vi "log analysis_gps.vi"() -> ()   [LabVIEW 2019] (continued)
\tsystem status\tnormal 2 27.800000 0 0\trobot status\t31.327624\t41.295864\t9.189700\t-0.525200\t0.456230\t-124.593983\t0.494000\t-0.009000\n\t\n15:51:51.4\tlog_raw\tgps_raw\t#INSPVAXA,USB3,0,48.0,FINESTEERING,2107,283929.450,02000000,471d,15824;INS_ALIGNMENT_COMPLETE,INS_RTKFIXED,37.37050057739,126.72118712143,9.1936,22.3000,-0.3554,-0.3037,0.0227,-0.396145969,0.312216334,214.731264498,0.4324,0.3037,0.5892,0.1125,0.0933,0.0800,0.0956,0.0998,5.2109,0f000001,0*e8b24b74\n\tsystem status\tnormal 2 27.800000 0 0\trobot status\t31.181031\t41.106514\t9.193600\t-0.396146\t0.312216\t-124.731264\t0.495000\t-0.003000\n\t\n15:51:51.9\tlog_raw\tgps_raw\t#INSPVAXA,USB3,0,48.0,FINESTEERING,2107,283929.950,02000000,471d,15824;INS_ALIGNMENT_COMPLETE,INS_RTKFIXED,37.37049890881,126.72118550326,9.1969,22.3000,-0.3488,-0.2994,0.0296,-0.491904024,0.536179959,214.904903866,0.4324,0.3037,0.5892,0.1125,0.0933,0.0800,0.0956,0.0998,5.2109,0f000001,0*ad87a7a5\n\tsystem status\tnormal 2 27.800000 0 0\trobot status\t31.037696\t40.921328\t9.196900\t-0.491904\t0.536180\t-124.904904\t0.491000\t-0.006000\n\t\n15:51:52.4\tlog_raw\tgps_raw\t#INSPVAXA,USB3,0,48.5,FINESTEERING,2107,283930.450,02000000,471d,15824;INS_ALIGNMENT_COMPLETE,INS_RTKFIXED,37.37049721050,126.72118386884,9.1995,22.3000,-0.3636,-0.2994,0.0018,-0.629398853,0.403170896,215.071222614,0.4325,0.3033,0.5894,0.1129,0.0937,0.0807,0.0956,0.0998,5.2121,0f000001,0*cd026204\n\tsystem status\tnormal 2 27.800000 0 0\trobot status\t30.892922\t40.732842\t9.199500\t-0.629399\t0.403171\t-125.071223\t0.499000\t-0.003000\n\t\n15:51:52.9\tlog_raw\tgps_raw\t#INSPVAXA,USB3,0,48.5,FINESTEERING,2107,283930.950,02000000,471d,15824;INS_ALIGNMENT_COMPLETE,INS_RTKFIXED,37.37049554136,126.72118223903,9.2033,22.3000,-0.3579,-0.3114,0.0267,-0.630465931,0.456383664,215.164754622,0.4325,0.3033,0.5894,0.1129,0.0937,0.0807,0.0956,0.0998,5.2121,0f000001,0*d7b4217a\n\tsystem status\tnormal 2 27.800000 0 0\trobot status\t30.748556\t40.547594\t9.203300\t-0.630466\t0.456384\t-125.164755\t0.497000\t-0.001000\n\t\n15:51:53.4\tlog_raw\tgps_raw\t#INSPVAXA,USB3,0,51.0,FINESTEERING,2107,283931.450,02000000,471d,15824;INS_ALIGNMENT_COMPLETE,INS_RTKFIXED,37.37049384282,126.72118058399,9.2075,22.3000,-0.3544,-0.2989,0.0161,-0.740038291,0.456521512,215.355756173,0.4326,0.3033,0.5897,0.1135,0.0944,0.0819,0.0956,0.0998,5.2130,0f000001,0*1b20caf7\n\tsystem status\tnormal 2 27.800000 0 0\trobot status\t30.601955\t40.359083\t9.207500\t-0.740038\t0.456522\t-125.355756\t0.493000\t-0.002000\n\t\n15:51:53.9\tlog_raw\tgps_raw\t#INSPVAXA,USB3,0,51.0,FINESTEERING,2107,283931.950,02000000,471d,15824;INS_ALIGNMENT_COMPLETE,INS_RTKFIXED,37.37049213218,126.72117889345,9.2111,22.3000,-0.3596,-0.3121,0.0183,-0.657813953,0.413680306,215.408958644,0.4326,0.3033,0.5897,0.1135,0.0944,0.0819,0.0956,0.0998,5.2130,0f000001,0*a46484af\n\tsystem status\tnormal 2 27.800000 0 0\trobot status\t30.452210\t40.169228\t9.211100\t-0.657814\t0.413680\t-125.408959\t0.501000\t0.009000\n\t\n15:51:54.4\tlog_raw\tgps_raw\t#INSPVAXA,USB3,0,50.0,FINESTEERING,2107,283932.450,02000000,471d,15824;INS_ALIGNMENT_COMPLETE,INS_RTKFIXED,37.37049046733,126.72117722659,9.2158,22.3000,-0.3473,-0.3092,0.0349,-0.590608670,0.319388706,215.361013781,0.4329,0.3036,0.5903,0.1143,0.0953,0.0834,0.0957,0.0998,5.2135,0f000001,0*5573a11c\n\tsystem status\tnormal 2 27.800000 0 0\trobot status\t30.304562\t39.984456\t9.215800\t-0.590609\t0.319389\t-125.361014\t0.489000\t0.004000\n\t\n15:51:54.9\tlog_raw\tgps_raw\t#INSPVAXA,USB3,0,50.0,FINESTEERING,2107,283932.950,02000000,471d,15824;INS_ALIGNMENT_COMPLETE,INS_RTKFIXED,37.37048877805,126.72117553421,9.2224,22.3000,-0.3576,-0.3071,0.0334,-0.545773763,0.550162659,215.419033819,0.4329,0.3036,0.5903,0.1143,0.0953,0.0834,0.0957,0.0998,5.2135,0f000001,0*06d0156c\n\tsystem status\tnormal 2 27.800000 0 0\trobot status\t30.154654\t39.796973\t9.222400\t-0.545774\t0.550163\t-125.419034\t0.505000\t-0.004000\n\t\n15:51:55.4\tlog_raw\tgps_raw\t#INSPVAXA,USB3,0,46.5,FINESTEERING,2107,283933.450,02000000,471d,15824;INS_ALIGNMENT_COMPLETE,INS_RTKFIXED,37.37048709327,126.72117385484,9.2273,22.3000,-0.3583,-0.3032,0.0201,-0.584226709,0.709789470,215.528367136,0.4335,0.3040,0.5913,0.1137,0.0945,0.0830,0.0957,0.0998,5.2139,0f000001,0*ba7d8e29\n\tsystem status\tnormal 2 27.800000 0 0\trobot status\t30.005898\t39.609989\t9.227300\t-0.584227\t0.709789\t-125.528367\t0.492000\t-0.004000\n\t\n15:51:55.9\tlog_raw\tgps_raw\t#INSPVAXA,USB3,0,46.5,FINESTEERING,2107,283933.950,02000000,471d,15824;INS_ALIGNMENT_COMPLETE,INS_RTKFIXED,37.37048540421,126.72117215519,9.2325,22.3000,-0.3686,-0.3092,0.0093,-0.663238373,0.676190653,215.463359493,0.4335,0.3040,0.5913,0.1137,0.0945,0.0830,0.0957,0.0998,5.2139,0f000001,0*5a7d9a35\n\tsystem status\tnormal 2 27.800000 0 0\trobot status\t29.855346\t39.422530\t9.232500\t-0.663238\t0.676191\t-125.463359\t0.494000\t0.014000\n\t\n15:51:56.4\tlog_raw\tgps_raw\t#INSPVAXA,USB3,0,51.5,FINESTEERING,2107,283934.450,02000000,471d,15824;INS_ALIGNMENT_COMPLETE,INS_RTKFIXED,37.37048375352,126.72117048246,9.2375,22.3000,-0.3734,-0.3205,0.0340,-0.435969106,0.945574003,215.391049185,0.4334,0.3041,0.5920,0.1131,0.0939,0.0826,0.0958,0.0998,5.2143,0f000001,0*bcbd8a70\n\tsystem status\tnormal 2 27.700000 0 0\trobot status\t29.707178\t39.239329\t9.237500\t-0.435969\t0.945574\t-125.391049\t0.482000\t0.004000\n\t\n15:51:56.9\tlog_raw\tgps_raw\t#INSPVAXA,USB3,0,51.5,FINESTEERING,2107,283934.950,02000000,471d,15824;INS_ALIGNMENT_COMPLETE,INS_RTKFIXED,37.37048205847,126.72116880230,9.2433,22.3000,-0.3752,-0.3030,0.0191,-0.551123480,0.797684003,215.136467002,0.4334,0.3041,0.5920,0.1131,0.0939,0.0826,0.0958,0.0998,5.2143,0f000001,0*2d6be551\n\tsystem status\tnormal 2 27.700000 0 0\trobot status\t29.558352\t39.051205\t9.243300\t-0.551123\t0.797684\t-125.136467\t0.596000\t-0.155000\n\t\n15:51:57.4\tlog_raw\tgps_raw\t\tsystem status\tnormal 2 27.700000 0 0\trobot status\t29.409840\t38.862241\t9.248200\t-0.605044\t0.730671\t-124.996837\t0.601000\t-0.133000\n\t\n15:51:57.9\tlog_raw\tgps_raw\t#INSPVAXA,USB3,0,49.0,FINESTEERING,2107,283935.950,02000000,471d,15824;INS_ALIGNMENT_COMPLETE,INS_RTKFIXED,37.37047866137,126.72116545098,9.2537,22.3000,-0.3697,-0.3129,0.0257,-0.409292319,0.632531125,214.781702011,0.4334,0.3038,0.5927,0.1127,0.0935,0.0821,0.0959,0.0999,5.2145,0f000001,0*763cf472\n\tsystem status\tnormal 2 27.700000 0 0\trobot status\t29.261498\t38.674180\t9.253700\t-0.409292\t0.632531\t-124.781702\t0.607000\t-0.165000\n\t\n15:51:58.4\tlog_raw\tgps_raw\t#INSPVAXA,USB3,0,48.0,FINESTEERING,2107,283936.450,02000000,471d,15824;INS_ALIGNMENT_COMPLETE,INS_RTKFIXED,37.37047695933,126.72116379842,9.2575,22.3000,-0.3601,-0.2905,0.0223,-0.510166928,0.275357051,214.549267942,0.4332,0.3032,0.5933,0.1122,0.0932,0.0817,0.0960,0.0999,5.2143,0f000001,0*907ae007\n\tsystem status\tnormal 2 27.800000 0 0\trobot status\t29.115117\t38.485281\t9.257500\t-0.510167\t0.275357\t-124.549268\t0.469000\t0.034000\n\t\n15:51:58.9\tlog_raw\tgps_raw\t#INSPVAXA,USB3,0,48.0,FINESTEERING,2107,283936.950,02000000,471d,15824;INS_ALIGNMENT_COMPLETE,INS_RTKFIXED,37.37047527853,126.72116215716,9.2617,22.3000,-0.3613,-0.3073,0.0319,-0.493749348,0.435637715,214.244212344,0.4332,0.3032,0.5933,0.1122,0.0932,0.0817,0.0960,0.0999,5.2143,0f000001,0*77c5d1d8\n\tsystem status\tnormal 2 27.700000 0 0\trobot status\t28.969737\t38.298738\t9.261700\t-0.493749\t0.435638\t-124.244212\t0.497000\t-0.002000\n\t\n15:51:59.4\tlog_raw\tgps_raw\t\tsystem status\tnormal 2 27.700000 0 0\trobot status\t28.825588\t38.110134\t9.265500\t-0.511173\t0.534188\t-124.033120\t0.472000\t0.046000\n\t\n15:51:59.9\tlog_raw\tgps_raw\t#INSPVAXA,USB3,0,48.5,FINESTEERING,2107,283937.950,02000000,471d,15824;INS_ALIGNMENT_COMPLETE,INS_RTKFIXED,37.37047189710,126.72115890646,9.2688,22.3000,-0.3586,-0.2934,0.0244,-0.533486904,0.671561834,213.833990455,0.4328,0.3028,0.5937,0.1126,0.0939,0.0822,0.0961,0.1000,5.2146,0f000001,0*9215f66d\n\tsystem status\tnormal 2 27.700000 0 0\trobot status\t28.681795\t37.923453\t9.268800\t-0.533487\t0.671562\t-123.833990\t0.581000\t-0.140000\n\t\n15:52:00.4\tlog_raw\tgps_raw\t#INSPVAXA,USB3,0,52.0,FINESTEERING,2107,283938.450,02000000,471d,15824;INS_ALIGNMENT_COMPLETE,INS_RTKFIXED,37.37047020437,126.72115727420,9.2725,22.3000,-0.3547,-0.3143,0.0241,-0.356445317,0.659835202,213.629028548,0.4325,0.3026,0.5940,0.1125,0.0937,0.0818,0.0961,0.1000,5.2151,0f000001,0*9a205bce\n\tsystem status\tnormal 2 27.700000 0 0\trobot status\t28.537212\t37.735586\t9.272500\t-0.356445\t0.659835\t-123.629029\t0.583000\t-0.116000\n\t\n15:52:00.9\tlog_raw\tgps_raw\t#INSPVAXA,USB3,0,52.0,FINESTEERING,2107,283938.950,02000000,471d,15824;INS_ALIGNMENT_COMPLETE,INS_RTKFIXED,37.37046851551,126.72115567512,9.2776,22.3000,-0.3685,-0.3042,0.0189,-0.419579821,0.629946557,213.500724202,0.4325,0.3026,0.5940,0.1125,0.0937,0.0818,0.0961,0.1000,5.2151,0f000001,0*4752d92c\n\tsystem status\tnormal 2 27.700000 0 0\trobot status\t28.395568\t37.548149\t9.277600\t-0.419580\t0.629947\t-123.500724\t0.485000\t0.015000\n\t\n15:52:01.4\tlog_raw\tgps_raw\t\tsystem status\tnormal 2 27.700000 0 0\trobot status\t28.253926\t37.357358\t9.281600\t-0.443483\t0.611878\t-123.340546\t0.425000\t0.109000\n\t\n15:52:01.9\tlog_raw\tgps_raw\t#INSPVAXA,USB3,0,49.5,FINESTEERING,2107,283939.950,02000000,471d,15824;INS_ALIGNMENT_COMPLETE,INS_RTKFIXED,37.37046510443,126.72115247371,9.2872,22.3000,-0.3830,-0.2927,0.0256,-0.146641459,0.857904302,213.119748571,0.4322,0.3028,0.5939,0.1123,0.0936,0.0813,0.0961,0.1000,5.2160,0f000001,0*783a43e7\n\tsystem status\tnormal 2 27.700000 0 0\trobot status\t28.111992\t37.169573\t9.287200\t-0.146641\t0.857904\t-123.119749\t0.474000\t0.054000\n\t\n15:52:02.4\tlog_raw\tgps_raw\t\tsystem status\tnormal 2 27.700000 0 0\trobot status\t27.970600\t36.974764\t9.290600\t-0.325735\t0.638972\t-122.993373\t0.461000\t0.048000\n\t\n15:52:02.9\tlog_raw\tgps_raw\t\tsystem status\tnormal 2 27.700000 0 0\trobot status\t27.830324\t36.785318\t9.296100\t-0.266199\t0.640898\t-122.924032\t0.551000\t-0.116000\n\t\n15:52:03.4\tlog_raw\tgps_raw\t\tsystem status\tnormal 2 27.700000 0 0\trobot status\t27.688734\t36.591289\t9.301700\t-0.187271\t0.545822\t-122.764321\t0.436000\t0.104000\n\t\n15:52:03.9\tlog_raw\tgps_raw\t#INSPVAXA,USB3,0,46.5,FINESTEERING,2107,283941.950,02000000,471d,15824;INS_ALIGNMENT_COMPLETE,INS_RTKFIXED,37.37045819174,126.72114613372,9.3070,22.3000,-0.3933,-0.3167,0.0134,-0.360308060,0.744674803,212.733059130,0.4319,0.3027,0.5939,0.1126,0.0939,0.0813,0.0961,0.1000,5.2180,0f000001,0*c8f7eb70\n\tsystem status\tnormal 2 27.700000 0 0\trobot status\t27.550407\t36.402372\t9.307000\t-0.360308\t0.744675\t-122.733059\t0.474000\t0.039000\n\t\n15:52:04.4\tlog_raw\tgps_raw\t\tsystem status\tnormal 2 27.700000 0 0\trobot status\t27.410560\t36.213742\t9.313200\t-0.347803\t0.936763\t-122.761264\t0.552000\t-0.093000\n\t\n15:52:04.9\tlog_raw\tgps_raw\t\tsystem status\tnormal 2 27.800000 0 0\trobot status\t27.265855\t36.018088\t9.318000\t-0.322107\t0.870470\t-122.818582\t0.497000\t-0.008000\n\t\n15:52:05.4\tlog_raw\tgps_raw\t\tsystem status\tnormal 2 27.800000 0 0\trobot status\t27.127089\t35.827108\t9.324800\t-0.465411\t0.650638\t-122.727039\t0.496000\t-0.002000\n\t\n15:52:05.9\tlog_raw\tgps_raw\t\tsystem status\tnormal 2 27.700000 0 0\trobot status\t26.989455\t35.638881\t9.330900\t-0.534193\t0.584046\t-122.759127\t0.497000\t-0.006000\n\t\n15:52:06.4\tlog_raw\tgps_raw\t#INSPVAXA,USB3,0,51.5,FINESTEERING,2107,283944.450,02000000,471d,15824;INS_ALIGNMENT_COMPLETE,INS_RTKFIXED,37.37044958989,126.72113821345,9.3358,22.3000,-0.3641,-0.3051,0.0226,-0.383976023,0.466369784,212.614223269,0.4320,0.3035,0.5933,0.1137,0.0952,0.0823,0.0960,0.1000,5.2226,0f000001,0*0b47cfbf\n\tsystem status\tnormal 2 27.700000 0 0\trobot status\t26.848842\t35.447702\t9.335800\t-0.383976\t0.466370\t-122.614223\t0.463000\t0.040000\n\t\n15:52:06.9\tlog_raw\tgps_raw\t\tsystem status\tnormal 2 27.800000 0 0\trobot status\t26.706802\t35.252989\t9.340400\t-0.677953\t0.353917\t-122.801534\t0.481000\t0.000000\n\t\n15:52:07.4\tlog_raw\tgps_raw\t\tsystem status\tnormal 2 27.800000 0 0\trobot status\t26.569227\t35.067797\t9.346800\t-0.848730\t0.734301\t-122.803165\t0.514000\t-0.011000\n\t\n15:52:07.9\tlog_raw\tgps_raw\t#INSPVAXA,USB3,0,51.0,FINESTEERING,2107,283945.950,02000000,471d,15824;INS_ALIGNMENT_COMPLETE,INS_RTKFIXED,37.37044449644,126.72113345903,9.3530,22.3000,-0.3492,-0.2810,0.0259,-0.492056173,0.868162173,212.637209572,0.4322,0.3030,0.5933,0.1133,0.0945,0.0819,0.0959,0.1000,5.2239,0f000001,0*fbf44ee4\n\tsystem status\tnormal 2 27.700000 0 0\trobot status\t26.427703\t34.882409\t9.353000\t-0.492056\t0.868162\t-122.637210\t0.452000\t0.049000\n\t\n15:52:08.4\tlog_raw\tgps_raw\t\tsystem status\tnormal 2 27.800000 0 0\trobot status\t26.286479\t34.688227\t9.357400\t-0.761292\t0.766320\t-122.659869\t0.412000\t0.105000\n\t\n15:52:08.9\tlog_raw\tgps_raw\t\tsystem status\tnormal 2 27.700000 0 0\trobot status\t26.147636\t34.500909\t9.364200\t-0.701421\t0.861484\t-122.585257\t0.534000\t-0.023000\n\t\n15:52:09.4\tlog_raw\tgps_raw\t\tsystem status\tnormal 2 27.700000 0 0\trobot status\t26.011706\t34.313477\t9.369900\t-0.696279\t0.838753\t-122.386827\t0.564000\t-0.107000\n\t\n15:52:09.9\tlog_raw\tgps_raw\t#INSPVAXA,USB3,0,50.5,FINESTEERING,2107,283947.950,02000000,471d,15824;INS_ALIGNMENT_COMPLETE,INS_RTKFIXED,37.37043763245,126.72112720109,9.3747,22.3000,-0.3517,-0.2756,0.0362,-0.981277004,0.835950889,212.295904790,0.4324,0.3035,0.5933,0.1126,0.0937,0.0812,0.0959,0.0999,5.2264,0f000001,0*ec5c30da\n\tsystem status\tnormal 2 27.700000 0 0\trobot status\t25.873385\t34.120613\t9.374700\t-0.981277\t0.835951\t-122.295905\t0.571000\t-0.133000\n\t\n15:52:10.4\tlog_raw\tgps_raw\t#INSPVAXA,USB3,0,51.0,FINESTEERING,2107,283948.450,02000000,471d,15824;INS_ALIGNMENT_COMPLETE,INS_RTKFIXED,37.37043588029,126.72112562917,9.3803,22.3000,-0.3710,-0.2973,0.0467,-0.738282510,0.795123885,212.189518726,0.4321,0.3032,0.5932,0.1125,0.0934,0.0808,0.0959,0.0999,5.2279,0f000001,0*ed2f12b7\n\tsystem status\tnormal 2 27.700000 0 0\trobot status\t25.734147\t33.926151\t9.380300\t-0.738283\t0.795124\t-122.189519\t0.472000\t0.031000\n\t\n15:52:10.9\tlog_raw\tgps_raw\t\tsystem status\tnormal 2 27.700000 0 0\trobot status\t25.599973\t33.733191\t9.383700\t-0.886852\t0.904015\t-122.033887\t0.432000\t0.043000\n\t\n15:52:11.4\tlog_raw\tgps_raw\t\tsystem status\tnormal 2 27.700000 0 0\trobot status\t25.470337\t33.549136\t9.388700\t-1.093921\t1.011067\t-121.839455\t0.530000\t-0.010000\n\t\n15:52:11.9\tlog_raw\tgps_raw\t\tsystem status\tnormal 2 27.700000 0 0\trobot status\t25.335389\t33.360450\t9.394100\t-1.032375\t1.131480\t-121.781321\t0.521000\t-0.025000\n\t\n15:52:12.4\tlog_raw\tgps_raw\t\tsystem status\tnormal 2 27.700000 0 0\trobot status\t25.200705\t33.165178\t9.396900\t-1.255987\t0.856864\t-121.737226\t0.412000\t0.093000\n\t\n15:52:12.9\tlog_raw\tgps_raw\t\tsystem status\tnormal 2 27.800000 0 0\trobot status\t25.063179\t32.968041\t9.400200\t-1.373882\t0.716125\t-121.740815\t0.489000\t0.008000\n\t\n15:52:13.4\tlog_raw\tgps_raw\t\tsystem status\tnormal 2 27.700000 0 0\trobot status\t24.930042\t32.776821\t9.404200\t-1.457285\t0.898088\t-121.763485\t0.513000\t-0.018000\n\t\n15:52:13.9\tlog_raw\tgps_raw\t\tsystem status\tnormal 2 27.700000 0 0\trobot status\t24.796204\t32.585371\t9.407800\t-1.429968\t0.916304\t-121.673053\t0.554000\t-0.095000\n\t\n15:52:14.4\tlog_raw\tgps_raw\t\tsystem status\tnormal 2 27.800000 0 0\trobot status\t24.658979\t32.385980\t9.412700\t-1.267755\t0.772140\t-121.641050\t0.484000\t0.003000\n\t\n15:52:14.9\tlog_raw\tgps_raw\t\tsystem status\tnormal 2 27.800000 0 0\trobot status\t24.521969\t32.187371\t9.418000\t-1.235594\t0.519604\t-121.693191\t0.505000\t-0.002000\n\t\n15:52:15.4\tlog_raw\tgps_raw\t#INSPVAXA,USB3,0,50.5,FINESTEERING,2107,283953.450,02008000,471d,15824;INS_ALIGNMENT_COMPLETE,INS_RTKFIXED,37.37041847684,126.72111045346,9.4216,22.3000,-0.3714,-0.2867,0.0304,-1.344882424,0.718506073,211.705510005,0.4322,0.3022,0.5921,0.1132,0.0948,0.0813,0.0958,0.0998,5.2323,0f000001,0*748620fd\n\tsystem status\tnormal 2 27.800000 0 0\trobot status\t24.389908\t31.994640\t9.421600\t-1.344882\t0.718506\t-121.705510\t0.472000\t0.003000\n\t\n15:52:15.9\tlog_raw\tgps_raw\t\tsystem status\tnormal 2 27.800000 0 0\trobot status\t24.254545\t31.800433\t9.427600\t-1.214573\t0.724221\t-121.552443\t0.434000\t0.105000\n\t\n15:52:16.4\tlog_raw\tgps_raw\t\tsystem status\tnormal 2 27.800000 0 0\trobot status\t24.123389\t31.605480\t9.431900\t-1.255225\t1.024369\t-121.591230\t0.507000\t-0.044000\n\t\n15:52:16.9\tlog_raw\tgps_raw\t\tsystem status\tnormal 2 27.800000 0 0\trobot status\t23.992248\t31.411533\t9.437800\t-1.153355\t1.047772\t-121.505044\t0.504000\t0.001000\n\t\n15:52:17.4\tlog_raw\tgps_raw\t\tsystem status\tnormal 2 27.800000 0 0\trobot status\t23.859344\t31.215363\t9.440900\t-1.186232\t0.986175\t-121.519494\t0.490000\t-0.004000\n\t\n15:52:17.9\tlog_raw\tgps_raw\t\tsystem status\tnormal 2 27.700000 0 0\trobot status\t23.728436\t31.021752\t9.445600\t-1.389175\t0.781643\t-121.489086\t0.530000\t-0.075000\n\t\n15:52:18.4\tlog_raw\tgps_raw\t\tsystem status\tnormal 2 27.800000 0 0\trobot status\t23.591855\t30.820735\t9.449300\t-1.217600\t0.468155\t-121.519724\t0.552000\t-0.126000\n\t\n15:52:18.9\tlog_raw\tgps_raw\t\tsystem status\tnormal 2 27.700000 0 0\trobot status\t23.460737\t30.626485\t9.453300\t-1.115461\t0.670083\t-121.424643\t0.514000\t-0.006000\n\t\n15:52:19.4\tlog_raw\tgps_raw\t\tsystem status\tnormal 2 27.800000 0 0\trobot status\t23.330451\t30.435925\t9.456900\t-1.173128\t0.702816\t-121.498714\t0.503000\t-0.006000\n\t\n15:52:19.9\tlog_raw\tgps_raw\t\tsystem status\tnormal 2 27.700000 0 0\trobot status\t23.195575\t30.239420\t9.460300\t-1.230379\t0.512986\t-121.529406\t0.488000\t-0.011000\n\t\n15:52:20.5\tlog_raw\tgps_raw\t\tsystem status\tnormal 2 27.800000 0 0\trobot status\t23.061335\t30.044020\t9.464000\t-1.179429\t0.256991\t-121.541413\t0.496000\t-0.001000\n\t\n15:52:20.9\tlog_raw\tgps_raw\t\tsystem status\tnormal 2 27.800000 0 0\trobot status\t22.928458\t29.852934\t9.468000\t-1.150379\t0.429055\t-121.647260\t0.501000\t-0.006000\n\t\n15:52:21.5\tlog_raw\tgps_raw\t\tsystem status\tnormal 2 27.800000 0 0\trobot status\t22.795869\t29.662698\t9.470800\t-1.064563\t0.694386\t-121.699241\t0.474000\t0.001000\n\t\n15:52:22.0\tlog_raw\tgps_raw\t\tsystem status\tnormal 2 27.800000 0 0\trobot status\t22.661364\t29.469936\t9.473100\t-1.073659\t0.626375\t-121.658714\t0.491000\t0.003000\n\t\n15:52:22.5\tlog_raw\tgps_raw\t\tsystem status\tnormal 2 27.700000 0 0\trobot status\t22.525625\t29.278657\t9.476100\t-0.877335\t0.478267\t-121.735223\t0.485000\t-0.006000\n\t\n15:52:23.0\tlog_raw\tgps_raw\t\tsystem status\tnormal 2 27.800000 0 0\trobot status\t22.392194\t29.090539\t9.480900\t-0.833361\t0.791650\t-121.726009\t0.498000\t0.004000\n\t\n15:52:23.5\tlog_raw\tgps_raw\t\tsystem status\tnormal 2 27.800000 0 0\trobot status\t22.255642\t28.895525\t9.483500\t-0.765592\t0.928080\t-121.763148\t0.486000\t0.000000\n\t\n15:52:24.0\tlog_raw\tgps_raw\t\tsystem status\tnormal 2 27.700000 0 0\trobot status\t22.119331\t28.704042\t9.485800\t-0.670231\t0.668228\t-121.847801\t0.497000\t-0.012000\n\t\n15:52:24.5\tlog_raw\tgps_raw\t\tsystem status\tnormal 2 27.800000 0 0\trobot status\t21.981741\t28.509725\t9.489500\t-0.624551\t0.073942\t-121.796723\t0.492000\t0.011000\n\t\n15:52:25.0\tlog_raw\tgps_raw\t\tsystem status\tnormal 2 27.800000 0 0\trobot status\t21.844037\t28.318712\t9.492000\t-0.576923\t0.033651\t-121.804660\t0.495000\t0.007000\n\t\n15:52:25.5\tlog_raw\tgps_raw\t\tsystem status\tnormal 2 27.800000 0 0\trobot status\t21.707876\t28.127417\t9.493300\t-0.622223\t0.440759\t-121.927597\t0.494000\t-0.003000\n\t\n15:52:26.0\tlog_raw\tgps_raw\t\tsystem status\tnormal 2 27.700000 0 0\trobot status\t21.569619\t27.937516\t9.495700\t-0.543209\t0.517434\t-121.947062\t0.504000\t-0.010000\n\t\n15:52:26.5\tlog_raw\tgps_raw\t\tsystem status\tnormal 2 27.700000 0 0\trobot status\t21.431241\t27.743852\t9.498300\t-0.685465\t0.256216\t-122.020582\t0.488000\t-0.006000\n\t\n15:52:27.0\tlog_raw\tgps_raw\t\tsystem status\tnormal 2 27.800000 0 0\trobot status\t21.294228\t27.556128\t9.502100\t-0.670214\t0.347415\t-122.023855\t0.502000\t-0.009000\n\t\n15:52:27.5\tlog_raw\tgps_raw\t\tsystem status\tnormal 2 27.700000 0 0\trobot status\t21.153779\t27.364656\t9.503100\t-0.519527\t0.304295\t-121.984980\t0.559000\t-0.124000\n\t\n15:52:28.0\tlog_raw\tgps_raw\t\tsystem status\tnormal 2 27.800000 0 0\trobot status\t21.016086\t27.176227\t9.504100\t-0.719402\t0.235059\t-122.001127\t0.492000\t0.001000\n\t\n15:52:28.5\tlog_raw\tgps_raw\t\tsystem status\tnormal 2 27.700000 0 0\trobot status\t20.878531\t26.986469\t9.506100\t-0.828158\t0.273130\t-122.012669\t0.587000\t-0.141000\n\t\n15:52:29.0\tlog_raw\tgps_raw\t\tsystem status\tnormal 2 27.800000 0 0\trobot status\t20.741483\t26.799887\t9.506900\t-0.659979\t0.265214\t-121.934855\t0.466000\t0.043000\n\t\n15:52:29.5\tlog_raw\tgps_raw\t\tsystem status\tnormal 2 27.700000 0 0\trobot status\t20.604716\t26.609502\t9.508600\t-0.644342\t0.257472\t-121.852697\t0.476000\t0.039000\n\t\n15:52:30.0\tlog_raw\tgps_raw\t\tsystem status\tnormal 2 27.700000 0 0\trobot status\t20.469072\t26.418926\t9.508900\t-0.749614\t0.593945\t-121.796478\t0.481000\t0.039000\n\t\n15:52:30.5\tlog_raw\tgps_raw\t\tsystem status\tnormal 2 27.700000 0 0\trobot status\t20.333556\t26.227367\t9.510000\t-0.543835\t0.297563\t-121.540523\t0.416000\t0.124000\n\t\n15:52:31.0\tlog_raw\tgps_raw\t\tsystem status\tnormal 2 27.700000 0 0\trobot status\t20.199795\t26.034837\t9.511600\t-0.785621\t0.173532\t-121.481353\t0.450000\t0.064000\n\t\n15:52:31.5\tlog_raw\tgps_raw\t\tsystem status\tnormal 2 27.700000 0 0\trobot status\t20.067953\t25.840147\t9.514500\t-1.001172\t0.384623\t-121.454994\t0.614000\t-0.169000\n\t\n15:52:32.0\tlog_raw\tgps_raw\t\tsystem status\tnormal 2 27.800000 0 0\trobot status\t19.934734\t25.647459\t9.516600\t-0.851666\t0.454143\t-121.346911\t0.463000\t0.047000\n\t\n15:52:32.5\tlog_raw\tgps_raw\t\tsystem status\tnormal 2 27.700000 0 0\trobot status\t19.804377\t25.452957\t9.519200\t-1.071150\t0.547562\t-121.301318\t0.435000\t0.085000\n\t\n15:52:33.0\tlog_raw\tgps_raw\t\tsystem status\tnormal 2 27.700000 0 0\trobot status\t19.673009\t25.258683\t9.523800\t-1.105328\t0.619486\t-121.308098\t0.447000\t0.063000\n\t\n15:52:33.5\tlog_raw\tgps_raw\t\tsystem status\tnormal 2 27.800000 0 0\trobot status\t19.540232\t25.063740\t9.526400\t-1.182351\t0.733962\t-121.333426\t0.485000\t-0.003000\n\t\n15:52:34.0\tlog_raw\tgps_raw\t\tsystem status\tnormal 2 27.800000 0 0\trobot status\t19.411134\t24.875078\t9.528800\t-1.286442\t0.715185\t-121.304058\t0.495000\t0.000000\n\t\n15:52:34.5\tlog_raw\tgps_raw\t\tsystem status\tnormal 2 27.800000 0 0\trobot status\t19.278347\t24.678981\t9.531500\t-1.283525\t0.654556\t-121.406468\t0.497000\t-0.005000\n\t\n15:52:35.0\tlog_raw\tgps_raw\t\tsystem status\tnormal 2 27.800000 0 0\trobot status\t19.147763\t24.486216\t9.533900\t-1.378909\t0.521127\t-121.420029\t0.491000\t0.004000\n\t\n15:52:35.5\tlog_raw\tgps_raw\t\tsystem status\tnormal 2 27.800000 0 0\trobot status\t19.016303\t24.290989\t9.537000\t-1.317253\t0.379457\t-121.478546\t0.498000\t-0.006000\n\t\n15:52:36.0\tlog_raw\tgps_raw\t\tsystem status\tnormal 2 27.800000 0 0\trobot status\t18.886502\t24.098579\t9.540700\t-1.338638\t0.856192\t-121.625080\t0.496000\t-0.006000\n\t\n15:52:36.5\tlog_raw\tgps_raw\t\tsystem status\tnormal 2 27.800000 0 0\trobot status\t18.754019\t23.900758\t9.542100\t-1.340291\t0.507125\t-121.700074\t0.485000\t-0.008000\n\t\n15:52:37.0\tlog_raw\tgps_raw\t\tsystem status\tnormal 2 27.800000 0 0\trobot status\t18.621506\t23.704544\t9.545500\t-1.313061\t0.261436\t-121.705567\t0.493000\t0.008000\n\t\n15:52:37.5\tlog_raw\tgps_raw\t#INSPVAXA,USB3,0,48.5,FINESTEERING,2107,283975.500,02000000,471d,15824;INS_ALIGNMENT_COMPLETE,INS_RTKFIXED,37.37034183103,126.72104365598,9.5499,22.3000,-0.3648,-0.2725,0.0197,-1.244402765,0.202153747,211.898676033,0.4326,0.3045,0.5916,0.1133,0.0944,0.0814,0.0956,0.0997,5.2502,0f000001,0*746e4bd4\n\tsystem status\tnormal 2 27.800000 0 0\trobot status\t18.473096\t23.488151\t9.549900\t-1.244403\t0.202154\t-121.898676\t0.495000\t-0.010000\n\t\n15:52:38.0\tlog_raw\tgps_raw\t\tsystem status\tnormal 2 27.800000 0 0\trobot status\t18.350843\t23.312662\t9.553000\t-1.206263\t0.263199\t-122.051256\t0.491000\t-0.009000\n\t\n15:52:38.5\tlog_raw\tgps_raw\t\tsystem status\tnormal 2 27.800000 0 0\trobot status\t18.216468\t23.120426\t9.555500\t-1.271150\t0.574983\t-122.189288\t0.498000\t-0.011000\n\t\n15:52:39.0\tlog_raw\tgps_raw\t\tsystem status\tnormal 2 27.800000 0 0\trobot status\t18.080960\t22.926749\t9.561100\t-1.389187\t0.579422\t-122.410225\t0.496000\t-0.013000\n\t\n15:52:39.5\tlog_raw\tgps_raw\t\tsystem status\tnormal 2 27.800000 0 0\trobot status\t17.942939\t22.733049\t9.563300\t-1.147991\t0.700768\t-122.538594\t0.492000\t-0.011000\n\t\n15:52:40.0\tlog_raw\tgps_raw\t\tsystem status\tnormal 2 27.800000 0 0\trobot status\t17.803710\t22.536669\t9.565200\t-1.298443\t0.511147\t-122.793110\t0.487000\t-0.011000\n\t\n15:52:40.5\tlog_raw\tgps_raw\t\tsystem status\tnormal 2 27.800000 0 0\trobot status\t17.664905\t22.344510\t9.568300\t-1.353209\t0.659517\t-123.144040\t0.495000\t-0.009000\n\t\n15:52:41.0\tlog_raw\tgps_raw\t#INSPVAXA,USB3,0,50.5,FINESTEERING,2107,283979.000,02000000,471d,15824;INS_ALIGNMENT_COMPLETE,INS_RTKFIXED,37.37032960177,126.72103274756,9.5709,22.3000,-0.3611,-0.2914,0.0231,-1.123681308,0.223311003,213.340300492,0.4324,0.3037,0.5929,0.1134,0.0946,0.0828,0.0957,0.0996,5.2509,0f000001,0*020bc469\n\tsystem status\tnormal 2 27.800000 0 0\trobot status\t17.506846\t22.130894\t9.570900\t-1.123681\t0.223311\t-123.340300\t0.500000\t-0.004000\n\t\n15:52:41.5\tlog_raw\tgps_raw\t\tsystem status\tnormal 2 27.800000 0 0\trobot status\t17.379163\t21.958115\t9.573200\t-1.115970\t0.134377\t-123.508090\t0.486000\t-0.016000\n\t\n15:52:42.0\tlog_raw\tgps_raw\t#INSPVAXA,USB3,0,51.5,FINESTEERING,2107,283980.000,02000000,471d,15824;INS_ALIGNMENT_COMPLETE,INS_RTKFIXED,37.37032615968,126.72102953721,9.5775,22.3000,-0.3586,-0.2940,0.0139,-1.097113995,0.335693778,213.663017986,0.4326,0.3036,0.5938,0.1129,0.0941,0.0824,0.0958,0.0997,5.2514,0f000001,0*6db47364\n\tsystem status\tnormal 2 27.800000 0 0\trobot status\t17.222479\t21.748875\t9.577500\t-1.097114\t0.335694\t-123.663018\t0.502000\t0.002000\n\t\n15:52:42.5\tlog_raw\tgps_raw\t\tsystem status\tnormal 2 27.800000 0 0\trobot status\t17.093887\t21.580111\t9.578800\t-0.918026\t0.521413\t-123.838402\t0.492000\t0.005000\n\t\n15:52:43.0\tlog_raw\tgps_raw\t\tsystem status\tnormal 2 27.700000 0 0\trobot status\t16.950688\t21.391310\t9.582700\t-0.952841\t0.713763\t-123.972927\t0.486000\t-0.001000\n\t\n15:52:43.5\tlog_raw\tgps_raw\t#INSPVAXA,USB3,0,49.5,FINESTEERING,2107,283981.500,02008000,471d,15824;INS_ALIGNMENT_COMPLETE,INS_RTKFIXED,37.37032104015,126.72102467256,9.5879,22.3000,-0.3441,-0.2878,0.0186,-1.054014794,0.825950094,214.092959020,0.4321,0.3029,0.5950,0.1124,0.0936,0.0820,0.0959,0.0998,5.2531,0f000001,0*2dd59142\n\tsystem status\tnormal 2 27.800000 0 0\trobot status\t16.791576\t21.180687\t9.587900\t-1.054015\t0.825950\t-124.092959\t0.497000\t0.000000\n\t\n15:52:44.0\tlog_raw\tgps_raw\t\tsystem status\tnormal 2 27.800000 0 0\trobot status\t16.659868\t21.011535\t9.592500\t-0.850377\t0.837656\t-124.143145\t0.505000\t0.000000\n\t\n15:52:44.5\tlog_raw\tgps_raw\t\tsystem status\tnormal 2 27.800000 0 0\trobot status\t16.515514\t20.822606\t9.597100\t-0.945917\t0.853906\t-124.283025\t0.488000\t0.001000\n\t\n15:52:45.0\tlog_raw\tgps_raw\t\tsystem status\tnormal 2 27.800000 0 0\trobot status\t16.370087\t20.635169\t9.601300\t-1.077017\t0.693727\t-124.268501\t0.491000\t0.006000\n\t\n15:52:45.5\tlog_raw\tgps_raw\t\tsystem status\tnormal 2 27.700000 0 0\trobot status\t16.225148\t20.447970\t9.608700\t-1.008323\t1.017097\t-124.284253\t0.498000\t0.013000\n\t\n15:52:46.0\tlog_raw\tgps_raw\t\tsystem status\tnormal 2 27.800000 0 0\trobot status\t16.077510\t20.257254\t9.613900\t-1.024239\t0.813005\t-124.416018\t0.492000\t-0.004000\n\t\n15:52:46.5\tlog_raw\tgps_raw\t\tsystem status\tnormal 2 27.700000 0 0\trobot status\t15.933277\t20.071786\t9.620400\t-1.025367\t1.027138\t-124.357430\t0.507000\t0.004000\n\t\n15:52:47.0\tlog_raw\tgps_raw\t\tsystem status\tnormal 2 27.800000 0 0\trobot status\t15.783833\t19.881373\t9.626500\t-1.072110\t0.851984\t-124.486261\t0.434000\t0.106000\n\t\n15:52:47.5\tlog_raw\tgps_raw\t\tsystem status\tnormal 2 27.700000 0 0\trobot status\t15.641666\t19.696698\t9.633700\t-1.226607\t0.779637\t-124.303756\t0.467000\t0.034000\n\t\n15:52:48.0\tlog_raw\tgps_raw\t#INSPVAXA,USB3,0,52.0,FINESTEERING,2107,283986.000,02000000,471d,15824;INS_ALIGNMENT_COMPLETE,INS_RTKFIXED,37.37030579801,126.72100988006,9.6428,22.3000,-0.3555,-0.3000,0.0366,-1.295250272,1.014100957,214.138979775,0.4311,0.3032,0.5948,0.1121,0.0935,0.0806,0.0960,0.0999,5.2589,0f000001,0*23ad1ff8\n\tsystem status\tnormal 2 27.700000 0 0\trobot status\t15.481281\t19.489047\t9.642800\t-1.295250\t1.014101\t-124.138980\t0.469000\t0.054000\n\t\n15:52:48.5\tlog_raw\tgps_raw\t\tsystem status\tnormal 2 27.700000 0 0\trobot status\t15.352376\t19.319414\t9.649100\t-1.266633\t1.285771\t-123.953225\t0.483000\t0.030000\n\t\n15:52:49.0\tlog_raw\tgps_raw\t#INSPVAXA,USB3,0,52.0,FINESTEERING,2107,283987.000,02000000,471d,15824;INS_ALIGNMENT_COMPLETE,INS_RTKFIXED,37.37030239327,126.72100663816,9.6587,22.3000,-0.3682,-0.2898,0.0587,-1.329893089,1.153647504,213.823414970,0.4310,0.3029,0.5945,0.1121,0.0935,0.0803,0.0960,0.0999,5.2604,0f000001,0*f674c8ef\n\tsystem status\tnormal 2 27.700000 0 0\trobot status\t15.194118\t19.111174\t9.658700\t-1.329893\t1.153648\t-123.823415\t0.412000\t0.111000\n\t\n15:52:49.5\tlog_raw\tgps_raw\t#INSPVAXA,USB3,0,49.5,FINESTEERING,2107,283987.500,02000000,471d,15824;INS_ALIGNMENT_COMPLETE,INS_RTKFIXED,37.37030066241,126.72100502191,9.6668,22.3000,-0.3610,-0.3081,0.0180,-1.422130124,0.889324413,213.618378707,0.4310,0.3029,0.5940,0.1122,0.0936,0.0801,0.0959,0.0999,5.2619,0f000001,0*76fbb7ae\n\tsystem status\tnormal 2 27.700000 0 0\trobot status\t15.050954\t18.919075\t9.666800\t-1.422130\t0.889324\t-123.618379\t0.608000\t-0.127000\n\t\n15:52:50.0\tlog_raw\tgps_raw\t#INSPVAXA,USB3,0,49.5,FINESTEERING,2107,283988.000,02000000,471d,15824;INS_ALIGNMENT_COMPLETE,INS_RTKFIXED,37.37029896329,126.72100339526,9.6748,22.3000,-0.3691,-0.2999,0.0388,-1.192200282,0.602579891,213.591513237,0.4310,0.3029,0.5940,0.1122,0.0936,0.0801,0.0959,0.0999,5.2619,0f000001,0*354c1358\n\tsystem status\tnormal 2 27.700000 0 0\trobot status\t14.906868\t18.730499\t9.674800\t-1.192200\t0.602580\t-123.591513\t0.596000\t-0.169000\n\t\n15:52:50.5\tlog_raw\tgps_raw\t\tsystem status\tnormal 2 27.700000 0 0\trobot status\t14.778303\t18.557917\t9.680600\t-1.210157\t0.717041\t-123.354039\t0.594000\t-0.161000\n\t\n15:52:51.0\tlog_raw\tgps_raw\t\tsystem status\tnormal 2 27.700000 0 0\trobot status\t14.634502\t18.365379\t9.685700\t-1.122354\t0.837113\t-123.253836\t0.420000\t0.122000\n\t\n15:52:51.5\tlog_raw\tgps_raw\t#INSPVAXA,USB3,0,48.5,FINESTEERING,2107,283989.500,02000000,471d,15824;INS_ALIGNMENT_COMPLETE,INS_RTKFIXED,37.37029378078,126.72099856141,9.6916,22.3000,-0.3611,-0.2878,0.0332,-0.977406801,0.664431366,213.036331796,0.4317,0.3028,0.5934,0.1135,0.0949,0.0816,0.0957,0.0998,5.2642,0f000001,0*80882a82\n\tsystem status\tnormal 2 27.700000 0 0\trobot status\t14.478693\t18.155321\t9.691600\t-0.977407\t0.664431\t-123.036332\t0.589000\t-0.154000\n\t\n15:52:52.0\tlog_raw\tgps_raw\t#INSPVAXA,USB3,0,48.5,FINESTEERING,2107,283990.000,02000000,471d,15824;INS_ALIGNMENT_COMPLETE,INS_RTKFIXED,37.37029204407,126.72099699457,9.6988,22.3000,-0.3771,-0.2894,0.0402,-1.247584491,0.667932801,212.987583360,0.4317,0.3028,0.5934,0.1135,0.0949,0.0816,0.0957,0.0998,5.2642,0f000001,0*cfed9a10\n\tsystem status\tnormal 2 27.700000 0 0\trobot status\t14.339905\t17.962573\t9.698800\t-1.247584\t0.667933\t-122.987583\t0.573000\t-0.113000\n\t\n15:52:52.5\tlog_raw\tgps_raw\t#INSPVAXA,USB3,0,50.0,FINESTEERING,2107,283990.500,02000000,471d,15824;INS_ALIGNMENT_COMPLETE,INS_RTKFIXED,37.37029029580,126.72099542809,9.7025,22.3000,-0.3670,-0.2925,0.0054,-1.144620935,0.833749283,212.845661627,0.4315,0.3031,0.5931,0.1131,0.0946,0.0813,0.0957,0.0998,5.2654,0f000001,0*19c2a41b\n\tsystem status\tnormal 2 27.700000 0 0\trobot status\t14.201149\t17.768543\t9.702500\t-1.144621\t0.833749\t-122.845662\t0.432000\t0.082000\n\t\n15:52:53.0\tlog_raw\tgps_raw\t#INSPVAXA,USB3,0,50.0,FINESTEERING,2107,283991.000,02000000,471d,15824;INS_ALIGNMENT_COMPLETE,INS_RTKFIXED,37.37028854245,126.72099383471,9.7082,22.3000,-0.3734,-0.2981,0.0505,-1.053794581,0.860705414,212.916628462,0.4315,0.3031,0.5931,0.1131,0.0946,0.0813,0.0957,0.0998,5.2654,0f000001,0*6cd9c21a\n\tsystem status\tnormal 2 27.800000 0 0\trobot status\t14.060010\t17.573948\t9.708200\t-1.053795\t0.860705\t-122.916628\t0.501000\t-0.012000\n\t\n15:52:53.5\tlog_raw\tgps_raw\t#INSPVAXA,USB3,0,50.0,FINESTEERING,2107,283991.500,02000000,471d,15824;INS_ALIGNMENT_COMPLETE,INS_RTKFIXED,37.37028678118,126.72099223881,9.7128,22.3000,-0.3905,-0.2870,0.0338,-1.308863276,0.828346639,212.947096436,0.4317,0.3031,0.5932,0.1128,0.0940,0.0810,0.0956,0.0998,5.2662,0f000001,0*9682182f\n\tsystem status\tnormal 2 27.800000 0 0\trobot status\t13.918648\t17.378474\t9.712800\t-1.308863\t0.828347\t-122.947096\t0.502000\t-0.013000\n\t\n15:52:54.0\tlog_raw\tgps_raw\t#INSPVAXA,USB3,0,50.0,FINESTEERING,2107,283992.000,02000000,471d,15824;INS_ALIGNMENT_COMPLETE,INS_RTKFIXED,37.37028506885,126.72099063831,9.7202,22.3000,-0.3587,-0.3008,0.0194,-1.224018986,0.834141555,212.863695719,0.4317,0.3031,0.5932,0.1128,0.0940,0.0810,0.0956,0.0998,5.2662,0f000001,0*43bde827\n\tsystem status\tnormal 2 27.800000 0 0\trobot status\t13.776878\t17.188432\t9.720200\t-1.224019\t0.834142\t-122.863696\t0.489000\t0.004000\n\t\n15:52:54.5\tlog_raw\tgps_raw\t#INSPVAXA,USB3,0,45.0,FINESTEERING,2107,283992.500,02000000,471d,15824;INS_ALIGNMENT_COMPLETE,INS_RTKFIXED,37.37028333459,126.72098904452,9.7257,22.3000,-0.3784,-0.2965,0.0443,-1.050562507,0.745679158,212.979675556,0.4319,0.3033,0.5933,0.1130,0.0942,0.0816,0.0956,0.0997,5.2672,0f000001,0*f6d38c7c\n\tsystem status\tnormal 2 27.700000 0 0\trobot status\t13.635703\t16.995956\t9.725700\t-1.050563\t0.745679\t-122.979676\t0.495000\t-0.016000\n\t\n15:52:55.0\tlog_raw\tgps_raw\t#INSPVAXA,USB3,0,45.0,FINESTEERING,2107,283993.000,02000000,471d,15824;INS_ALIGNMENT_COMPLETE,INS_RTKFIXED,37.37028161694,126.72098748507,9.7305,22.3000,-0.3588,-0.2835,0.0413,-1.341951739,0.883295300,213.030480888,0.4319,0.3033,0.5933,0.1130,0.0942,0.0816,0.0956,0.0997,5.2672,0f000001,0*8bfaad14\n\tsystem status\tnormal 2 27.800000 0 0\trobot status\t13.497569\t16.805324\t9.730500\t-1.341952\t0.883295\t-123.030481\t0.493000\t-0.004000\n\t\n15:52:55.5\tlog_raw\tgps_raw\t#INSPVAXA,USB3,0,49.0,FINESTEERING,2107,283993.500,02000000,471d,15824;INS_ALIGNMENT_COMPLETE,INS_RTKFIXED,37.37027987729,126.72098589860,9.7339,22.3000,-0.3886,-0.3118,0.0118,-1.186705860,0.635599144,213.040521206,0.4318,0.3035,0.5934,0.1127,0.0938,0.0813,0.0956,0.0997,5.2685,0f000001,0*5b9abbf8\n\tsystem status\tnormal 2 27.700000 0 0\trobot status\t13.357042\t16.612250\t9.733900\t-1.186706\t0.635599\t-123.040521\t0.501000\t0.000000\n\t\n15:52:56.0\tlog_raw\tgps_raw\t#INSPVAXA,USB3,0,49.0,FINESTEERING,2107,283994.000,02000000,471d,15824;INS_ALIGNMENT_COMPLETE,INS_RTKFIXED,37.37027813856,126.72098430051,9.7386,22.3000,-0.3794,-0.2983,0.0413,-1.126640911,0.427805755,213.093758144,0.4318,0.3035,0.5934,0.1127,0.0938,0.0813,0.0956,0.0997,5.2685,0f000001,0*e42dd86e\n\tsystem status\tnormal 2 27.800000 0 0\trobot status\t13.215486\t16.419278\t9.738600\t-1.126641\t0.427806\t-123.093758\t0.484000\t-0.002000\n\t\n15:52:56.5\tlog_raw\tgps_raw\t#INSPVAXA,USB3,0,41.5,FINESTEERING,2107,283994.500,02000000,471d,15824;INS_ALIGNMENT_COMPLETE,INS_RTKFIXED,37.37027639241,126.72098271837,9.7433,22.3000,-0.3724,-0.2941,0.0395,-1.023992417,0.392331965,213.143460080,0.4318,0.3036,0.5935,0.1130,0.0944,0.0820,0.0956,0.0997,5.2698,0f000001,0*0337d50d\n\tsystem status\tnormal 2 27.800000 0 0\trobot status\t13.075343\t16.225482\t9.743300\t-1.023992\t0.392332\t-123.143460\t0.499000\t-0.008000\n\t\n15:52:57.0\tlog_raw\tgps_raw\t#INSPVAXA,USB3,0,41.5,FINESTEERING,2107,283995.000,02000000,471d,15824;INS_ALIGNMENT_COMPLETE,INS_RTKFIXED,37.37027465637,126.72098113948,9.7472,22.3000,-0.3708,-0.2998,0.0087,-1.064940932,0.419900141,213.213279076,0.4318,0.3036,0.5935,0.1130,0.0944,0.0820,0.0956,0.0997,5.2698,0f000001,0*335ddb23\n\tsystem status\tnormal 2 27.800000 0 0\trobot status\t12.935487\t16.032809\t9.747200\t-1.064941\t0.419900\t-123.213279\t0.500000\t0.005000\n\t\n15:52:57.5\tlog_raw\tgps_raw\t#INSPVAXA,USB3,0,49.5,FINESTEERING,2107,283995.500,02000000,471d,15824;INS_ALIGNMENT_COMPLETE,INS_RTKFIXED,37.37027293232,126.72097957470,9.7494,22.3000,-0.3727,-0.2928,0.0273,-1.114629129,0.419021826,213.334562050,0.4319,0.3032,0.5939,0.1127,0.0939,0.0817,0.0957,0.0997,5.2708,0f000001,0*bec96f91\n\tsystem status\tnormal 2 27.800000 0 0\trobot status\t12.796881\t15.841466\t9.749400\t-1.114629\t0.419022\t-123.334562\t0.493000\t0.006000\n\t\n15:52:58.0\tlog_raw\tgps_raw\t#INSPVAXA,USB3,0,49.5,FINESTEERING,2107,283996.000,02000000,471d,15824;INS_ALIGNMENT_COMPLETE,INS_RTKFIXED,37.37027121924,126.72097799640,9.7538,22.3000,-0.3785,-0.2972,0.0344,-0.912805448,0.531088142,213.375963340,0.4319,0.3032,0.5939,0.1127,0.0939,0.0817,0.0957,0.0997,5.2708,0f000001,0*e0fc992c\n\tsystem status\tnormal 2 27.800000 0 0\trobot status\t12.657078\t15.651341\t9.753800\t-0.912805\t0.531088\t-123.375963\t0.507000\t0.000000\n\t\n15:52:58.5\tlog_raw\tgps_raw\t#INSPVAXA,USB3,0,48.5,FINESTEERING,2107,283996.500,02000000,471d,15824;INS_ALIGNMENT_COMPLETE,INS_RTKFIXED,37.37026950707,126.72097642523,9.7575,22.3000,-0.3790,-0.2971,0.0045,-1.031000712,0.442701672,213.487798192,0.4317,0.3031,0.5940,0.1124,0.0936,0.0813,0.0957,0.0997,5.2719,0f000001,0*6ebbd163\n\tsystem status\tnormal 2 27.800000 0 0\trobot status\t12.517907\t15.461316\t9.757500\t-1.031001\t0.442702\t-123.487798\t0.494000\t-0.006000\n\t\n15:52:59.0\tlog_raw\tgps_raw\t#INSPVAXA,USB3,0,48.5,FINESTEERING,2107,283997.000,02000000,471d,15824;INS_ALIGNMENT_COMPLETE,INS_RTKFIXED,37.37026778904,126.72097482944,9.7613,22.3000,-0.3776,-0.3087,0.0370,-1.077110117,0.533414002,213.644467670,0.4317,0.3031,0.5940,0.1124,0.0936,0.0813,0.0957,0.0997,5.2719,0f000001,0*eda6f981\n\tsystem status\tnormal 2 27.800000 0 0\trobot status\t12.376554\t15.270642\t9.761300\t-1.077110\t0.533414\t-123.644468\t0.495000\t-0.007000\n\t\n15:52:59.5\tlog_raw\tgps_raw\t#INSPVAXA,USB3,0,51.5,FINESTEERING,2107,283997.500,02000000,471d,15824;INS_ALIGNMENT_COMPLETE,INS_RTKFIXED,37.37026610502,126.72097322741,9.7652,22.3000,-0.3735,-0.2926,0.0418,-0.879042002,0.635388403,213.712940335,0.4318,0.3033,0.5943,0.1122,0.0934,0.0810,0.0958,0.0998,5.2733,0f000001,0*c5914784\n\tsystem status\tnormal 2 27.800000 0 0\trobot status\t12.234649\t15.083742\t9.765200\t-0.879042\t0.635388\t-123.712940\t0.498000\t-0.006000\n\t\n15:53:00.0\tlog_raw\tgps_raw\t#INSPVAXA,USB3,0,51.5,FINESTEERING,2107,283998.000,02000000,471d,15824;INS_ALIGNMENT_COMPLETE,INS_RTKFIXED,37.37026439172,126.72097159305,9.7705,22.3000,-0.3793,-0.3043,0.0231,-0.804340415,0.481108177,213.810502820,0.4318,0.3033,0.5943,0.1122,0.0934,0.0810,0.0958,0.0998,5.2733,0f000001,0*97086bfc\n\tsystem status\tnormal 2 27.700000 0 0\trobot status\t12.089880\t14.893592\t9.770500\t-0.804340\t0.481108\t-123.810503\t0.505000\t0.000000\n\t\n15:53:00.5\tlog_raw\tgps_raw\t#INSPVAXA,USB3,0,51.0,FINESTEERING,2107,283998.500,02000000,471d,15824;INS_ALIGNMENT_COMPLETE,INS_RTKFIXED,37.37026268780,126.72097001383,9.7729,22.3000,-0.3715,-0.3065,0.0247,-0.969252583,0.581649669,213.913706075,0.4317,0.3034,0.5943,0.1125,0.0938,0.0813,0.0958,0.0998,5.2748,0f000001,0*e268e54b\n\tsystem status\tnormal 2 27.800000 0 0\trobot 
